vi "VISJS Viewer.vi"(4 "Extra Scripts":string, 5 "FileDependency In":map{path, T1}(c390), 6 "Options":string, 7 "OpenWebBrowser(False)":bool, 8 "error in":errorcluster, 9 "Embedd VISJS Librarya in HTMl File(False)":bool, 10 "HTMLFilePath":path, 11 "LibraryDependency":map{path, T3}(c390)) -> (0 "error out":errorcluster, 3 "HTMLFileContent":string)   [LabVIEW 2020, in "VISJS Viewer.lvlib"] (continued)
0,#385380);border:1px solid #14334b;border-radius:50%;box-shadow:0 0 1px 0 #111927;filter:progid:DXImageTransform.Microsoft.gradient(startColorstr=\"#3876c2\",endColorstr=\"#385380\",GradientType=0);height:17px;margin-top:-7px;width:17px}input.vis-configuration.vis-config-range:focus{outline:none}input.vis-configuration.vis-config-range:focus::-webkit-slider-runnable-track{background:#9d9d9d;background:-moz-linear-gradient(top,#9d9d9d 0,#c8c8c8 99%);background:-webkit-gradient(linear,left top,left bottom,color-stop(0,#9d9d9d),color-stop(99%,#c8c8c8));background:-webkit-linear-gradient(top,#9d9d9d,#c8c8c8 99%);background:-o-linear-gradient(top,#9d9d9d 0,#c8c8c8 99%);background:-ms-linear-gradient(top,#9d9d9d 0,#c8c8c8 99%);background:linear-gradient(180deg,#9d9d9d 0,#c8c8c8 99%);filter:progid:DXImageTransform.Microsoft.gradient(startColorstr=\"#9d9d9d\",endColorstr=\"#c8c8c8\",GradientType=0)}input.vis-configuration.vis-config-range::-moz-range-track{background:#dedede;background:-moz-linear-gradient(top,#dedede 0,#c8c8c8 99%);background:-webkit-gradient(linear,left top,left bottom,color-stop(0,#dedede),color-stop(99%,#c8c8c8));background:-webkit-linear-gradient(top,#dedede,#c8c8c8 99%);background:-o-linear-gradient(top,#dedede 0,#c8c8c8 99%);background:-ms-linear-gradient(top,#dedede 0,#c8c8c8 99%);background:linear-gradient(180deg,#dedede 0,#c8c8c8 99%);border:1px solid #999;border-radius:3px;box-shadow:0 0 3px 0 #aaa;filter:progid:DXImageTransform.Microsoft.gradient(startColorstr=\"#dedede\",endColorstr=\"#c8c8c8\",GradientType=0);height:10px;width:300px}input.vis-configuration.vis-config-range::-moz-range-thumb{background:#385380;border:none;border-radius:50%;height:16px;width:16px}input.vis-configuration.vis-config-range:-moz-focusring{outline:1px solid #fff;outline-offset:-1px}input.vis-configuration.vis-config-range::-ms-track{background:transparent;border-color:transparent;border-width:6px 0;color:transparent;height:5px;width:300px}input.vis-configuration.vis-config-range::-ms-fill-lower{background:#777;border-radius:10px}input.vis-configuration.vis-config-range::-ms-fill-upper{background:#ddd;border-radius:10px}input.vis-configuration.vis-config-range::-ms-thumb{background:#385380;border:none;border-radius:50%;height:16px;width:16px}input.vis-configuration.vis-config-range:focus::-ms-fill-lower{background:#888}input.vis-configuration.vis-config-range:focus::-ms-fill-upper{background:#ccc}.vis-configuration-popup{background:rgba(57,76,89,.85);border:2px solid #f2faff;border-radius:4px;color:#fff;font-size:14px;height:30px;line-height:30px;position:absolute;text-align:center;-webkit-transition:opacity .3s ease-in-out;-moz-transition:opacity .3s ease-in-out;transition:opacity .3s ease-in-out;width:150px}.vis-configuration-popup:after,.vis-configuration-popup:before{border:solid transparent;content:\" \";height:0;left:100%;pointer-events:none;position:absolute;top:50%;width:0}.vis-configuration-popup:after{border-color:rgba(136,183,213,0) rgba(136,183,213,0) rgba(136,183,213,0) rgba(57,76,89,.85);border-width:8px;margin-top:-8px}.vis-configuration-popup:before{border-color:rgba(194,225,245,0) rgba(194,225,245,0) rgba(194,225,245,0) #f2faff;border-width:12px;margin-top:-12px}');_e(\"div.vis-tooltip{background-color:#f5f4ed;border:1px solid #808074;-moz-border-radius:3px;-webkit-border-radius:3px;border-radius:3px;box-shadow:3px 3px 10px rgba(0,0,0,.2);color:#000;font-family:verdana;font-size:14px;padding:5px;pointer-events:none;position:absolute;visibility:hidden;white-space:nowrap;z-index:5}\");var Ke={exports:{}};!function(g){function t(g){if(g)return function(g){for(var A in t.prototype)g[A]=t.prototype[A];return g}(g)}g.exports=t,t.prototype.on=t.prototype.addEventListener=function(g,t){return this._callbacks=this._callbacks||{},(this._callbacks[\"$\"+g]=this._callbacks[\"$\"+g]||[]).push(t),this},t.prototype.once=function(g,t){function A(){this.off(g,A),t.apply(this,arguments)}return A.fn=t,this.on(g,A),this},t.prototype.off=t.prototype.removeListener=t.prototype.removeAllListeners=t.prototype.removeEventListener=function(g,t){if(this._callbacks=this._callbacks||{},0==arguments.length)return this._callbacks={},this;var A,e=this._callbacks[\"$\"+g];if(!e)return this;if(1==arguments.length)return delete this._callbacks[\"$\"+g],this;for(var C=0;C<e.length;C++)if((A=e[C])===t||A.fn===t){e.splice(C,1);break}return 0===e.length&&delete this._callbacks[\"$\"+g],this},t.prototype.emit=function(g){this._callbacks=this._callbacks||{};for(var t=new Array(arguments.length-1),A=this._callbacks[\"$\"+g],e=1;e<arguments.length;e++)t[e-1]=arguments[e];if(A){e=0;for(var C=(A=A.slice(0)).length;e<C;++e)A[e].apply(this,t)}return this},t.prototype.listeners=function(g){return this._callbacks=this._callbacks||{},this._callbacks[\"$\"+g]||[]},t.prototype.hasListeners=function(g){return!!this.listeners(g).length}}(Ke);var He=A(Ke.exports),Xe={};Xe[dt(\"toStringTag\")]=\"z\";var Je,qe,$e,gC=\"[object z]\"===String(Xe),tC=gC,AC=O,eC=y,CC=dt(\"toStringTag\"),IC=Object,iC=\"Arguments\"===eC(function(){return arguments}()),oC=tC?eC:function(g){var t,A,e;return void 0===g?\"Undefined\":null===g?\"Null\":\"string\"==typeof(A=function(g,t){try{return g[t]}catch(g){}}(t=IC(g),CC))?A:iC?eC(t):\"Object\"===(e=eC(t))&&AC(t.callee)?\"Arguments\":e},nC=oC,rC=String,sC=function(g){if(\"Symbol\"===nC(g))throw new TypeError(\"Cannot convert a Symbol value to a string\");return rC(g)},aC=u,dC=PA,hC=sC,lC=K,cC=aC(\"\".charAt),uC=aC(\"\".charCodeAt),pC=aC(\"\".slice),fC=function(g){return function(t,A){var e,C,I=hC(lC(t)),i=dC(A),o=I.length;return i<0||i>=o?g?\"\":void 0:(e=uC(I,i))<55296||e>56319||i+1===o||(C=uC(I,i+1))<56320||C>57343?g?cC(I,i):e:g?pC(I,i,i+2):C-56320+(e-55296<<10)+65536}},vC={codeAt:fC(!1),charAt:fC(!0)},yC=O,mC=C.WeakMap,bC=yC(mC)&&/native code/.test(String(mC)),wC=et,kC=Ug(\"keys\"),xC=function(g){return kC[g]||(kC[g]=wC(g))},EC=bC,OC=C,TC=gg,DC=uA,NC=qg,RC=Wg,PC=xC,MC=UA,BC=\"Object already initialized\",zC=OC.TypeError,SC=OC.WeakMap;if(EC||RC.state){var ZC=RC.state||(RC.state=new SC);ZC.get=ZC.get,ZC.has=ZC.has,ZC.set=ZC.set,Je=function(g,t){if(ZC.has(g))throw new zC(BC);return t.facade=g,ZC.set(g,t),t},qe=function(g){return ZC.get(g)||{}},$e=function(g){return ZC.has(g)}}else{var FC=PC(\"state\");MC[FC]=!0,Je=function(g,t){if(NC(g,FC))throw new zC(BC);return t.facade=g,DC(g,FC,t),t},qe=function(g){return NC(g,FC)?g[FC]:{}},$e=function(g){return NC(g,FC)}}var GC={set:Je,get:qe,has:$e,enforce:function(g){return $e(g)?qe(g):Je(g,{})},getterFor:function(g){return function(t){var A;if(!TC(t)||(A=qe(t)).type!==g)throw new zC(\"Incompatible receiver, \"+g+\" required\");return A}}},jC=D,LC=qg,VC=Function.prototype,YC=jC&&Object.getOwnPropertyDescriptor,WC=LC(VC,\"name\"),QC={EXISTS:WC,PROPER:WC&&\"something\"===function(){}.name,CONFIGURABLE:WC&&(!jC||jC&&YC(VC,\"name\").configurable)},UC={},_C=D,KC=qt,HC=Jt,XC=AA,JC=J,qC=Ae;UC.f=_C&&!KC?Object.defineProperties:function(g,t){XC(g);for(var A,e=JC(t),C=qC(t),I=C.length,i=0;I>i;)HC.f(g,A=C[i++],e[A]);return g};var $C,gI=ig(\"document\",\"documentElement\"),tI=AA,AI=UC,eI=$A,CI=UA,II=gI,iI=Et,oI=\"prototype\",nI=\"script\",rI=xC(\"IE_PROTO\"),sI=function(){},aI=function(g){return\"<\"+nI+\">\"+g+\"</\"+nI+\">\"},dI=function(g){g.write(aI(\"\")),g.close();var t=g.parentWindow.Object;return g=null,t},hI=function(){try{$C=new ActiveXObject(\"htmlfile\")}catch(g){}var g,t,A;hI=\"undefined\"!=typeof document?document.domain&&$C?dI($C):(t=iI(\"iframe\"),A=\"java\"+nI+\":\",t.style.display=\"none\",II.appendChild(t),t.src=String(A),(g=t.contentWindow.document).open(),g.write(aI(\"document.F=Object\")),g.close(),g.F):dI($C);for(var e=eI.length;e--;)delete hI[oI][eI[e]];return hI()};CI[rI]=!0;var lI,cI,uI,pI=Object.create||function(g,t){var A;return null!==g?(sI[oI]=tI(g),A=new sI,sI[oI]=null,A[rI]=g):A=hI(),void 0===t?A:AI.f(A,t)},fI=!I((function(){function g(){}return g.prototype.constructor=null,Object.getPrototypeOf(new g)!==g.prototype})),vI=qg,yI=O,mI=Hg,bI=fI,wI=xC(\"IE_PROTO\"),kI=Object,xI=kI.prototype,EI=bI?kI.getPrototypeOf:function(g){var t=mI(g);if(vI(t,wI))return t[wI];var A=t.constructor;return yI(A)&&t instanceof A?A.prototype:t instanceof kI?xI:null},OI=uA,TI=function(g,t,A,e){return e&&e.enumerable?g[t]=A:OI(g,t,A),g},DI=I,NI=O,RI=gg,PI=pI,MI=EI,BI=TI,zI=dt(\"iterator\"),SI=!1;[].keys&&(\"next\"in(uI=[].keys())?(cI=MI(MI(uI)))!==Object.prototype&&(lI=cI):SI=!0);var ZI=!RI(lI)||DI((function(){var g={};return lI[zI].call(g)!==g}));NI((lI=ZI?{}:PI(lI))[zI])||BI(lI,zI,(function(){return this}));var FI={IteratorPrototype:lI,BUGGY_SAFARI_ITERATORS:SI},GI=oC,jI=gC?{}.toString:function(){return\"[object \"+GI(this)+\"]\"},LI=gC,VI=Jt.f,YI=uA,WI=qg,QI=jI,UI=dt(\"toStringTag\"),_I=function(g,t,A,e){if(g){var C=A?g:g.prototype;WI(C,UI)||VI(C,UI,{configurable:!0,value:t}),e&&!LI&&YI(C,\"toString\",QI)}},KI={},HI=FI.IteratorPrototype,XI=pI,JI=G,qI=_I,$I=KI,gi=function(){return this},ti=u,Ai=Rg,ei=O,Ci=String,Ii=TypeError,ii=function(g,t,A){try{return ti(Ai(Object.getOwnPropertyDescriptor(g,t)[A]))}catch(g){}},oi=AA,ni=function(g){if(\"object\"==typeof g||ei(g))return g;throw new Ii(\"Can't set \"+Ci(g)+\" as a prototype\")},ri=Object.setPrototypeOf||(\"__proto__\"in{}?function(){var g,t=!1,A={};try{(g=ii(Object.prototype,\"__proto__\",\"set\"))(A,[]),t=A instanceof Array}catch(g){}return function(A,e){return oi(A),ni(e),t?g(A,e):A.__proto__=e,A}}():void 0),si=TA,ai=P,di=QC,hi=function(g,t,A,e){var C=t+\" Iterator\";return g.prototype=XI(HI,{next:JI(+!e,A)}),qI(g,C,!1,!0),$I[C]=gi,g},li=EI,ci=_I,ui=TI,pi=KI,fi=FI,vi=di.PROPER,yi=fi.BUGGY_SAFARI_ITERATORS,mi=dt(\"iterator\"),bi=\"keys\",wi=\"values\",ki=\"entries\",xi=function(){return this},Ei=function(g,t,A,e,C,I,i){hi(A,t,e);var o,n,r,s=function(g){if(g===C&&c)return c;if(!yi&&g&&g in h)return h[g];switch(g){case bi:case wi:case ki:return function(){return new A(this,g)}}return function(){return new A(this)}},a=t+\" Iterator\",d=!1,h=g.prototype,l=h[mi]||h[\"@@iterator\"]||C&&h[C],c=!yi&&l||s(C),u=\"Array\"===t&&h.entries||l;if(u&&(o=li(u.call(new g)))!==Object.prototype&&o.next&&(ci(o,a,!0,!0),pi[a]=xi),vi&&C===wi&&l&&l.name!==wi&&(d=!0,c=function(){return ai(l,this)}),C)if(n={values:s(wi),keys:I?c:s(bi),entries:s(ki)},i)for(r in n)(yi||d||!(r in h))&&ui(h,r,n[r]);else si({target:t,proto:!0,forced:yi||d},n);return i&&h[mi]!==c&&ui(h,mi,c,{name:C}),pi[t]=c,n},Oi=function(g,t){return{value:g,done:t}},Ti=vC.charAt,Di=sC,Ni=GC,Ri=Ei,Pi=Oi,Mi=\"String Iterator\",Bi=Ni.set,zi=Ni.getterFor(Mi);Ri(String,\"String\",(function(g){Bi(this,{type:Mi,string:Di(g),index:0})}),(function(){var g,t=zi(this),A=t.string,e=t.index;return e>=A.length?Pi(void 0,!0):(g=Ti(A,e),t.index+=g.length,Pi(g,!1))}));var Si=P,Zi=AA,Fi=Bg,Gi=function(g,t,A){var e,C;Zi(g);try{if(!(e=Fi(g,\"return\"))){if(\"throw\"===t)throw A;return A}e=Si(e,g)}catch(g){C=!0,e=g}if(\"throw\"===t)throw A;if(C)throw e;return Zi(e),A},ji=AA,Li=Gi,Vi=KI,Yi=dt(\"iterator\"),Wi=Array.prototype,Qi=function(g){return void 0!==g&&(Vi.Array===g||Wi[Yi]===g)},Ui=O,_i=Wg,Ki=u(Function.toString);Ui(_i.inspectSource)||(_i.inspectSource=function(g){return Ki(g)});var Hi=_i.inspectSource,Xi=u,Ji=I,qi=O,$i=oC,go=Hi,to=function(){},Ao=[],eo=ig(\"Reflect\",\"construct\"),Co=/^\\s*(?:class|function)\\b/,Io=Xi(Co.exec),io=!Co.test(to),oo=function(g){if(!qi(g))return!1;try{return eo(to,Ao,g),!0}catch(g){return!1}},no=function(g){if(!qi(g))return!1;switch($i(g)){case\"AsyncFunction\":case\"GeneratorFunction\":case\"AsyncGeneratorFunction\":return!1}try{return io||!!Io(Co,go(g))}catch(g){return!0}};no.sham=!0;var ro=!eo||Ji((function(){var g;return oo(oo.call)||!oo(Object)||!oo((function(){g=!0}))||g}))?no:oo,so=bt,ao=Jt,ho=G,lo=function(g,t,A){var e=so(t);e in g?ao.f(g,e,ho(0,A)):g[e]=A},co=oC,uo=Bg,po=Q,fo=KI,vo=dt(\"iterator\"),yo=function(g){if(!po(g))return uo(g,vo)||uo(g,\"@@iterator\")||fo[co(g)]},mo=P,bo=Rg,wo=AA,ko=Og,xo=yo,Eo=TypeError,Oo=function(g,t){var A=arguments.length<2?xo(g):t;if(bo(A))return wo(mo(A,g));throw new Eo(ko(g)+\" is not iterable\")},To=Xt,Do=P,No=Hg,Ro=function(g,t,A,e){try{return e?t(ji(A)[0],A[1]):t(A)}catch(t){Li(g,\"throw\",t)}},Po=Qi,Mo=ro,Bo=jA,zo=lo,So=Oo,Zo=yo,Fo=Array,Go=dt(\"iterator\"),jo=!1;try{var Lo=0,Vo={next:function(){return{done:!!Lo++}},return:function(){jo=!0}};Vo[Go]=function(){return this},Array.from(Vo,(function(){throw 2}))}catch(g){}var Yo=function(g,t){try{if(!t&&!jo)return!1}catch(g){return!1}var A=!1;try{var e={};e[Go]=function(){return{next:function(){return{done:A=!0}}}},g(e)}catch(g){}return A},Wo=function(g){var t=No(g),A=Mo(this),e=arguments.length,C=e>1?arguments[1]:void 0,I=void 0!==C;I&&(C=To(C,e>2?arguments[2]:void 0));var i,o,n,r,s,a,d=Zo(t),h=0;if(!d||this===Fo&&Po(d))for(i=Bo(t),o=A?new this(i):Fo(i);i>h;h++)a=I?C(t[h],h):t[h],zo(o,h,a);else for(s=(r=So(t,d)).next,o=A?new this:[];!(n=Do(s,r)).done;h++)a=I?Ro(r,C,[n.value,h],!0):n.value,zo(o,h,a);return o.length=h,o};TA({target:\"Array\",stat:!0,forced:!Yo((function(g){Array.from(g)}))},{from:Wo});var Qo=tg.Array.from,Uo=A(Qo),_o=J,Ko=KI,Ho=GC;Jt.f;var Xo=Ei,Jo=Oi,qo=\"Array Iterator\",$o=Ho.set,gn=Ho.getterFor(qo);Xo(Array,\"Array\",(function(g,t){$o(this,{type:qo,target:_o(g),index:0,kind:t})}),(function(){var g=gn(this),t=g.target,A=g.kind,e=g.index++;if(!t||e>=t.length)return g.target=void 0,Jo(void 0,!0);switch(A){case\"keys\":return Jo(e,!1);case\"values\":return Jo(t[e],!1)}return Jo([e,t[e]],!1)}),\"values\"),Ko.Arguments=Ko.Array;var tn=yo,An={CSSRuleList:0,CSSStyleDeclaration:0,CSSValueList:0,ClientRectList:0,DOMRectList:0,DOMStringList:0,DOMTokenList:1,DataTransferItemList:0,FileList:0,HTMLAllCollection:0,HTMLCollection:0,HTMLFormElement:0,HTMLSelectElement:0,MediaList:0,MimeTypeArray:0,NamedNodeMap:0,NodeList:1,PaintRequestList:0,Plugin:0,PluginArray:0,SVGLengthList:0,SVGNumberList:0,SVGPathSegList:0,SVGPointList:0,SVGStringList:0,SVGTransformList:0,SourceBufferList:0,StyleSheetList:0,TextTrackCueList:0,TextTrackList:0,TouchList:0},en=C,Cn=oC,In=uA,on=KI,nn=dt(\"toStringTag\");for(var rn in An){var sn=en[rn],an=sn&&sn.prototype;an&&Cn(an)!==nn&&In(an,nn,rn),on[rn]=on.Array}var dn=tn,hn=A(dn),ln=A(dn);function cn(g,t){if(!(g instanceof t))throw new TypeError(\"Cannot call a class as a function\")}var un={exports:{}},pn=TA,fn=D,vn=Jt.f;pn({target:\"Object\",stat:!0,forced:Object.defineProperty!==vn,sham:!fn},{defineProperty:vn});var yn=tg.Object,mn=un.exports=function(g,t,A){return yn.defineProperty(g,t,A)};yn.defineProperty.sham&&(mn.sham=!0);var bn=un.exports,wn=bn,kn=A(wn),xn=y,En=Array.isArray||function(g){return\"Array\"===xn(g)},On=TypeError,Tn=function(g){if(g>9007199254740991)throw On(\"Maximum allowed index exceeded\");return g},Dn=En,Nn=ro,Rn=gg,Pn=dt(\"species\"),Mn=Array,Bn=function(g){var t;return Dn(g)&&(t=g.constructor,(Nn(t)&&(t===Mn||Dn(t.prototype))||Rn(t)&&null===(t=t[Pn]))&&(t=void 0)),void 0===t?Mn:t},zn=function(g,t){return new(Bn(g))(0===t?0:t)},Sn=I,Zn=cg,Fn=dt(\"species\"),Gn=function(g){return Zn>=51||!Sn((function(){var t=[];return(t.constructor={})[Fn]=function(){return{foo:1}},1!==t[g](Boolean).foo}))},jn=TA,Ln=I,Vn=En,Yn=gg,Wn=Hg,Qn=jA,Un=Tn,_n=lo,Kn=zn,Hn=Gn,Xn=cg,Jn=dt(\"isConcatSpreadable\"),qn=Xn>=51||!Ln((function(){var g=[];return g[Jn]=!1,g.concat()[0]!==g})),$n=function(g){if(!Yn(g))return!1;var t=g[Jn];return void 0!==t?!!t:Vn(g)};jn({target:\"Array\",proto:!0,arity:1,forced:!qn||!Hn(\"concat\")},{concat:function(g){var t,A,e,C,I,i=Wn(this),o=Kn(i,0),n=0;for(t=-1,e=arguments.length;t<e;t++)if($n(I=-1===t?i:arguments[t]))for(C=Qn(I),Un(n+C),A=0;A<C;A++,n++)A in I&&_n(o,n,I[A]);else Un(n+1),_n(o,n++,I);return o.length=n,o}});var gr={},tr=qA,Ar=$A.concat(\"length\",\"prototype\");gr.f=Object.getOwnPropertyNames||function(g){return tr(g,Ar)};var er={},Cr=SA,Ir=jA,ir=lo,or=Array,nr=Math.max,rr=function(g,t,A){for(var e=Ir(g),C=Cr(t,e),I=Cr(void 0===A?e:A,e),i=or(nr(I-C,0)),o=0;C<I;C++,o++)ir(i,o,g[C]);return i.length=o,i},sr=y,ar=J,dr=gr.f,hr=rr,lr=\"object\"==typeof window&&window&&Object.getOwnPropertyNames?Object.getOwnPropertyNames(window):[];er.f=function(g){return lr&&\"Window\"===sr(g)?function(g){try{return dr(g)}catch(g){return hr(lr)}}(g):dr(ar(g))};var cr=Jt,ur=function(g,t,A){return cr.f(g,t,A)},pr={},fr=dt;pr.f=fr;var vr=tg,yr=qg,mr=pr,br=Jt.f,wr=function(g){var t=vr.Symbol||(vr.Symbol={});yr(t,g)||br(t,g,{value:mr.f(g)})},kr=P,xr=ig,Er=dt,Or=TI,Tr=function(){var g=xr(\"Symbol\"),t=g&&g.prototype,A=t&&t.valueOf,e=Er(\"toPrimitive\");t&&!t[e]&&Or(t,e,(function(g){return kr(A,this)}),{arity:1})},Dr=Xt,Nr=W,Rr=Hg,Pr=jA,Mr=zn,Br=u([].push),zr=function(g){var t=1===g,A=2===g,e=3===g,C=4===g,I=6===g,i=7===g,o=5===g||I;return function(n,r,s,a){for(var d,h,l=Rr(n),c=Nr(l),u=Dr(r,s),p=Pr(c),f=0,v=a||Mr,y=t?v(n,p):A||i?v(n,0):void 0;p>f;f++)if((o||f in c)&&(h=u(d=c[f],f,l),g))if(t)y[f]=h;else if(h)switch(g){case 3:return!0;case 5:return d;case 6:return f;case 2:Br(y,d)}else switch(g){case 4:return!1;case 7:Br(y,d)}return I?-1:e||C?C:y}},Sr={forEach:zr(0),map:zr(1),filter:zr(2),some:zr(3),every:zr(4),find:zr(5),findIndex:zr(6),filterReject:zr(7)},Zr=TA,Fr=C,Gr=P,jr=u,Lr=D,Vr=vg,Yr=I,Wr=qg,Qr=og,Ur=AA,_r=J,Kr=bt,Hr=sC,Xr=G,Jr=pI,qr=Ae,$r=gr,gs=er,ts=ee,As=T,es=Jt,Cs=UC,Is=M,is=TI,os=ur,ns=Ug,rs=UA,ss=et,as=dt,ds=pr,hs=wr,ls=Tr,cs=_I,us=GC,ps=Sr.forEach,fs=xC(\"hidden\"),vs=\"Symbol\",ys=\"prototype\",ms=us.set,bs=us.getterFor(vs),ws=Object[ys],ks=Fr.Symbol,xs=ks&&ks[ys],Es=Fr.RangeError,Os=Fr.TypeError,Ts=Fr.QObject,Ds=As.f,Ns=es.f,Rs=gs.f,Ps=Is.f,Ms=jr([].push),Bs=ns(\"symbols\"),zs=ns(\"op-symbols\"),Ss=ns(\"wks\"),Zs=!Ts||!Ts[ys]||!Ts[ys].findChild,Fs=function(g,t,A){var e=Ds(ws,t);e&&delete ws[t],Ns(g,t,A),e&&g!==ws&&Ns(ws,t,e)},Gs=Lr&&Yr((function(){return 7!==Jr(Ns({},\"a\",{get:function(){return Ns(this,\"a\",{value:7}).a}})).a}))?Fs:Ns,js=function(g,t){var A=Bs[g]=Jr(xs);return ms(A,{type:vs,tag:g,description:t}),Lr||(A.description=t),A},Ls=function(g,t,A){g===ws&&Ls(zs,t,A),Ur(g);var e=Kr(t);return Ur(A),Wr(Bs,e)?(A.enumerable?(Wr(g,fs)&&g[fs][e]&&(g[fs][e]=!1),A=Jr(A,{enumerable:Xr(0,!1)})):(Wr(g,fs)||Ns(g,fs,Xr(1,{})),g[fs][e]=!0),Gs(g,e,A)):Ns(g,e,A)},Vs=function(g,t){Ur(g);var A=_r(t),e=qr(A).concat(Us(A));return ps(e,(function(t){Lr&&!Gr(Ys,A,t)||Ls(g,t,A[t])})),g},Ys=function(g){var t=Kr(g),A=Gr(Ps,this,t);return!(this===ws&&Wr(Bs,t)&&!Wr(zs,t))&&(!(A||!Wr(this,t)||!Wr(Bs,t)||Wr(this,fs)&&this[fs][t])||A)},Ws=function(g,t){var A=_r(g),e=Kr(t);if(A!==ws||!Wr(Bs,e)||Wr(zs,e)){var C=Ds(A,e);return!C||!Wr(Bs,e)||Wr(A,fs)&&A[fs][e]||(C.enumerable=!0),C}},Qs=function(g){var t=Rs(_r(g)),A=[];return ps(t,(function(g){Wr(Bs,g)||Wr(rs,g)||Ms(A,g)})),A},Us=function(g){var t=g===ws,A=Rs(t?zs:_r(g)),e=[];return ps(A,(function(g){!Wr(Bs,g)||t&&!Wr(ws,g)||Ms(e,Bs[g])})),e};Vr||(ks=function(){if(Qr(xs,this))throw new Os(\"Symbol is not a constructor\");var g=arguments.length&&void 0!==arguments[0]?Hr(arguments[0]):void 0,t=ss(g),A=function(g){this===ws&&Gr(A,zs,g),Wr(this,fs)&&Wr(this[fs],t)&&(this[fs][t]=!1);var e=Xr(1,g);try{Gs(this,t,e)}catch(g){if(!(g instanceof Es))throw g;Fs(this,t,e)}};return Lr&&Zs&&Gs(ws,t,{configurable:!0,set:A}),js(t,g)},is(xs=ks[ys],\"toString\",(function(){return bs(this).tag})),is(ks,\"withoutSetter\",(function(g){return js(ss(g),g)})),Is.f=Ys,es.f=Ls,Cs.f=Vs,As.f=Ws,$r.f=gs.f=Qs,ts.f=Us,ds.f=function(g){return js(as(g),g)},Lr&&os(xs,\"description\",{configurable:!0,get:function(){return bs(this).description}})),Zr({global:!0,constructor:!0,wrap:!0,forced:!Vr,sham:!Vr},{Symbol:ks}),ps(qr(Ss),(function(g){hs(g)})),Zr({target:vs,stat:!0,forced:!Vr},{useSetter:function(){Zs=!0},useSimple:function(){Zs=!1}}),Zr({target:\"Object\",stat:!0,forced:!Vr,sham:!Lr},{create:function(g,t){return void 0===t?Jr(g):Vs(Jr(g),t)},defineProperty:Ls,defineProperties:Vs,getOwnPropertyDescriptor:Ws}),Zr({target:\"Object\",stat:!0,forced:!Vr},{getOwnPropertyNames:Qs}),ls(),cs(ks,vs),rs[fs]=!0;var _s=vg&&!!Symbol.for&&!!Symbol.keyFor,Ks=TA,
